vi "DistanceSensor SonarReflectionsUpdate Event Example.vi"() -> ()   [LabVIEW 2012, in "Phidget Distance Sensor.lvlib"]
uses:
  <instrlib>/Phidgets/Phidget Distance Sensor/Phidget Distance Sensor.lvlib
  <instrlib>/Phidgets/Phidget Distance Sensor/Public/DistanceSensorStart.vi
  <instrlib>/Phidgets/Phidget Distance Sensor/Public/DistanceSensorClose.vi
  <instrlib>/Phidgets/Phidget Common/Phidget Common.lvlib
panel:
  out "Amplitudes":u32[](array[numeric])
  out "Distances":u32[](array[numeric])
  out "Count":u32
  in  "stop":bool
  out "Serial Number Return":i32
  in  "Device Info":T1={"Serial Number"=-1, "Channel"=0, "Port"=0}
  out "error out":errorcluster
  # "Be sure to use this stop button to stop the program.\nIf you use the \"Abort Execution\" button, you will\nneed to use PhidgetResetLibrary.vi or restart Labview \nin order for any Phidgets to work."
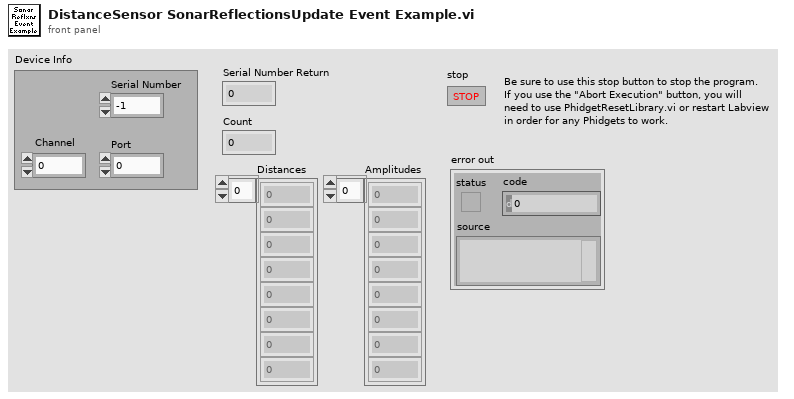
[diagram p1: front panel]
types:
  T1 = cluster{"Serial Number":i32, "Channel":i32, "Port":i32}
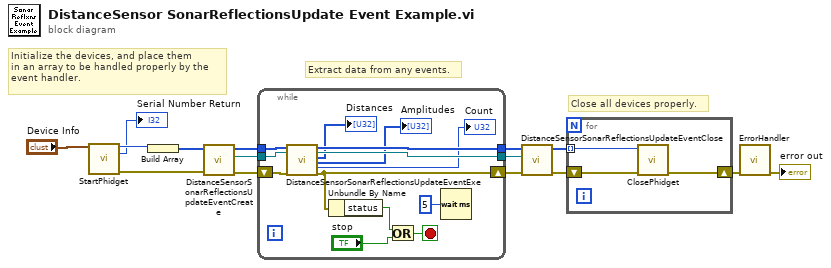
[diagram p0: block diagram]
diagram:
  # "Close all devices properly."
  # "Extract data from any events."
  # "Initialize the devices, and place them\nin an array to be handled properly by the\nevent handler."
  n1 = call-poly <instrlib>:"StartPhidget.vi"("Device Info"="Device Info") -> ("Phidget ID"=w5:u64, "Serial Number Return"=→"Serial Number Return":i32, "error out"=w2:errorcluster)  [unwired: 11 in, 1 out]
  n2 = Build Array(w5) -> (w15:u64[])
  n3 = call <instrlib>:"DistanceSensorSonarReflectionsUpdateEventCreate.vi"("error in (no error)"=w2, "Devices In"=w15) -> ("error out"=w8:errorcluster, "Event Registration Refnum"=w13:refnum<event-registration>, "Devices Out"=w14:u64[])  [unwired: 7 in]
  n4 = while {
    tunnel: w14 -> [w28]
    tunnel: w13 -> [w23]
    tunnel: [w27] -> w10
    shift-right: [w22] -> w9
    shift-left: w8 -> [w26]
    tunnel: [w24] -> w3
    stop <- w21 stop-if-true
    n5 = call <instrlib>:"DistanceSensorSonarReflectionsUpdateEventExe.vi"("Devices In"=w28, "Event Registration Refnum In"=w23, "error in (no error)"=w26) -> ("Devices Out"=w24:u64[], "Event Registration Refnum Out"=w27:refnum<event-registration>, "Distances"=→"Distances":u32[], "Amplitudes"=→"Amplitudes":u32[], "Count"=→"Count":u32, "error out"=w22:errorcluster)  [unwired: 8 in, 3 out]
    n6 = Unbundle By Name(w22) -> ("status"=w19:bool)
    n7 = Or(x=w19, y="stop") -> (x .or. y?=w21:bool)
    n8 = Wait (ms)(milliseconds to wait=u32 5) -> ()  [unwired: 1 out]
  }
  n9 = call <instrlib>:"DistanceSensorSonarReflectionsUpdateEventClose.vi"("error in (no error)"=w9, "Event Registration Refnum In"=w10, "Devices In"=w3) -> ("error out"=w6:errorcluster, "Devices Out"=w4:u64[])  [unwired: 7 in]
  n10 = for {
    tunnel: w4 -> [w29] mode=indexing
    shift-right: [w31] -> w12
    shift-left: w6 -> [w30]
    n11 = call-poly <instrlib>:"ClosePhidget.vi"("error in"=w30, "Device In"=w29) -> ("error out"=w31:errorcluster)  [unwired: 9 in]
  }
  n12 = call <instrlib>:"ErrorHandler.vi"("error in"=w12) -> ("error out"=→"error out":errorcluster)  [unwired: 9 in, 1 out]
